vi "Main.vi"(10 "Port Number":i16=4 min=0 max=20, 11 "Module Admin":refnum<class "Delacor_lib_QMH_Module Admin.lvclass">) -> ()   [LabVIEW 2020, in "Ophir Power Meter.lvlib"]
doc: "This template is based off of the Queued Message Handler design pattern and the Queued Message Handler project template that ships with LabVIEW.\n\nThe main difference is that the queue is private to this module and communication between modules is performed via Broadcast and Request events.\n\nRequest events are wrapped in public API methods and are handled in the Event Handling Loop (EHL) of this VI. Any module can register for Broadcast events sent by this module. The EHL generates messages based on user interface actions.\n\nThe Message Handling Loop (MHL) processes messages generated by the EHL, or by other messages. The messages are string values, so new messages can be added easily to the Message Cases case structure in the MHL. Each message cluster can also provide an optional value for Message Data, which is a variant that can be converted to whatever message-specific data is required.\n_____\nBased on Delacor QMH Project Template 5.0.0.82."
uses:
  Ophir Power Meter.lvlib
  <vilib>/Delacor/Delacor QMH/Libraries/Module Admin_class/Delacor_lib_QMH_Module Admin.lvclass
  Module Data--cluster.ctl
  Stop Argument--cluster.ctl
  <vilib>/Delacor/Delacor QMH/Libraries/Message Queue_class/Delacor_lib_QMH_Message Queue.lvclass/Delacor_lib_QMH_Message Queue.ctl
  <vilib>/Delacor/Delacor QMH/Libraries/Module Admin_class/Delacor_lib_QMH_Module Admin.lvclass/Delacor_lib_QMH_Module Admin.ctl
  Get Power Value Argument--cluster.ctl
  Get Power Value (Reply Payload)--cluster.ctl
  Select Range Argument--cluster.ctl
  Get Range Info Argument--cluster.ctl
  Get Range Info (Reply Payload)--cluster.ctl
  <vilib>/Utility/miscctls.llb/LVPointTypeDef.ctl
  <vilib>/Delacor/Delacor QMH/Libraries/Message Queue_class/Delacor_lib_QMH_Enqueue Message (Single).vi
  <vilib>/Delacor/Delacor QMH/Libraries/Module Admin_class/Delacor_lib_QMH_Get External Launch.vi
  <vilib>/Utility/error.llb/Error Cluster From Error Code.vi
  <vilib>/ErrorRing/Error Ring.xnode
  <vilib>/Delacor/Delacor QMH/Libraries/Message Queue_class/Delacor_lib_QMH_Message Queue.lvclass
panel:
  in  "Range":u16(ring)
  out "Power Value":dbl
  out "Units":string
  out "OK ?":bool
  out "Instrument Info":string[](array[string])
  out "error out":errorcluster
  out "Status":string
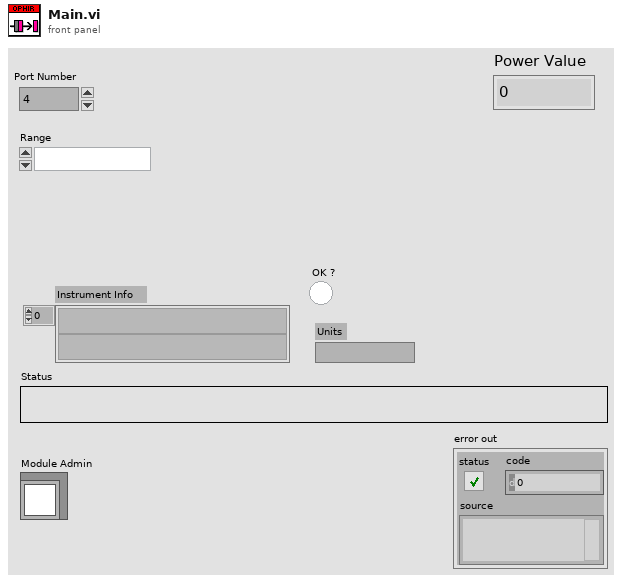
[diagram p1: front panel]
types:
  T1 = typedef "Ophir Power Meter.lvlib/Request Events--cluster.ctl" = cluster{"Stop Module":refnum<user-event>, "Show Panel":refnum<user-event>, "Hide Panel":refnum<user-event>, "Get Module Execution Status":refnum<user-event>, "Show Diagram":refnum<user-event>, "Get Power Value":refnum<user-event>, "Select Range":refnum<user-event>, "Get Range Info":refnum<user-event>}
  T2 = typedef "Ophir Power Meter.lvlib/Module Data--cluster.ctl" = cluster{"Status":string, "Visa Session":refnum<visa-resource-name>, "Range Info":cluster{"Strings Array":string[], "Symbols Array":i32[], "First Index":i32}}
  T3 = enum32{"invalid lock state", "Not Locked", "Locked (No Password)", "Password-protected"}
  T4 = typedef "Ophir Power Meter.lvlib/Stop Argument--cluster.ctl" = cluster{"Origin":string, "Exit via Stop Module Req?":bool, "Wait for Module to stop?":bool}
  T5 = typedef "Ophir Power Meter.lvlib/Get Power Value Argument--cluster.ctl" = cluster{"Wait Notifier":refnum<notifier>, "wait for reply":bool}
  T6 = typedef "Ophir Power Meter.lvlib/Select Range Argument--cluster.ctl" = cluster{"Range Number":i32}
  T7 = typedef "Ophir Power Meter.lvlib/Get Range Info Argument--cluster.ctl" = cluster{"Wait Notifier":refnum<notifier>, "wait for reply":bool}
  T8 = typedef "LVPointTypeDef.ctl" = cluster{"Horizontal":i16, "Vertical":i16}
  T9 = enum32{"Invalid", "Standard", "Closed", "Hidden", "Minimized", "Maximized"}
  T10 = typedef "Ophir Power Meter.lvlib/Get Power Value (Reply Payload)--cluster.ctl" = cluster{"Power Value":dbl, "Get Power Value_error":errorcluster}
  T11 = typedef "Ophir Power Meter.lvlib/Get Range Info (Reply Payload)--cluster.ctl" = cluster{"Range Info":cluster{"Strings Array":string[], "Symbols Array":i32[], "First Index":i32}, "Get Range Info_error":errorcluster}
  T12 = cluster{"Strings Array":string[], "Symbols Array":i32[], "First Index":i32}
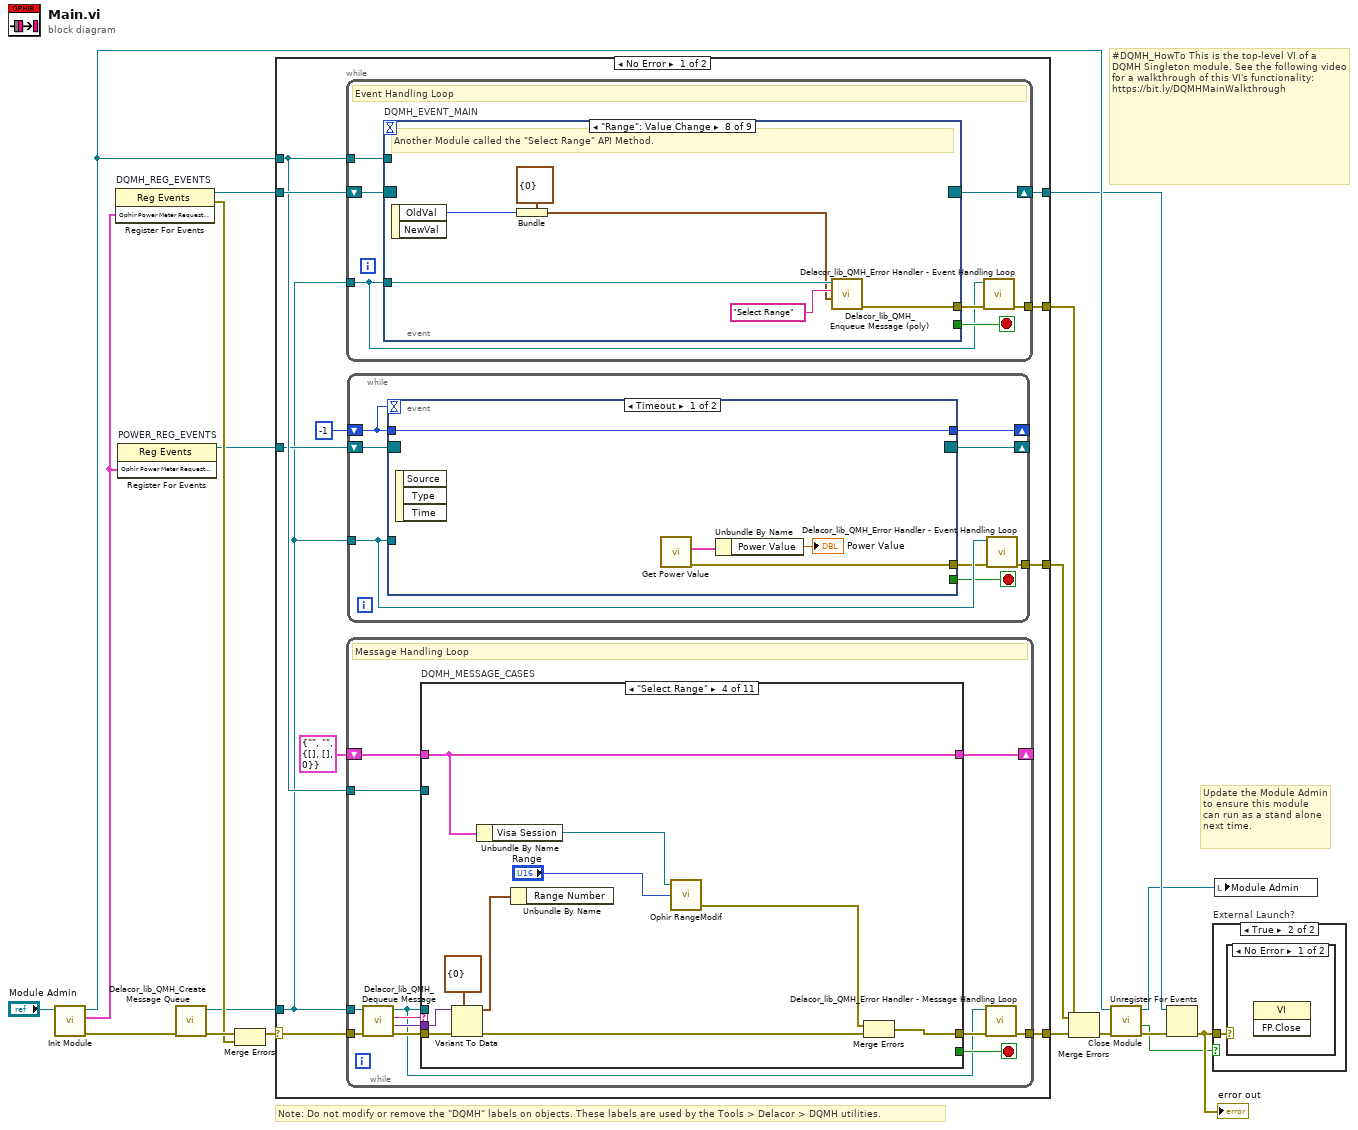
[diagram p0: block diagram]
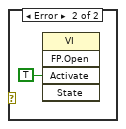
[diagram p3: hidden frame]
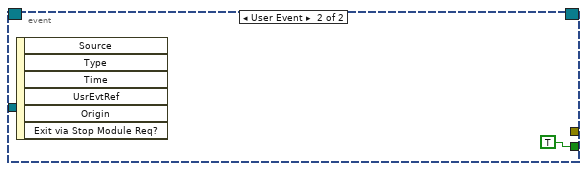
[diagram p4: hidden frame]
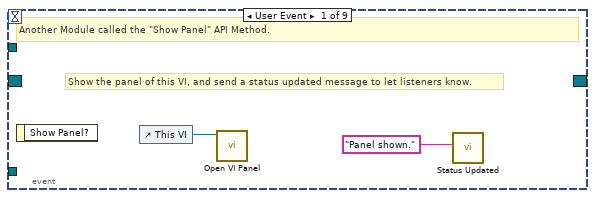
[diagram p5: hidden frame]
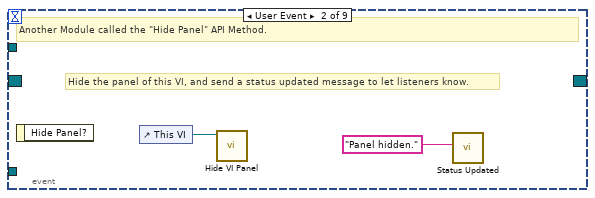
[diagram p6: hidden frame]
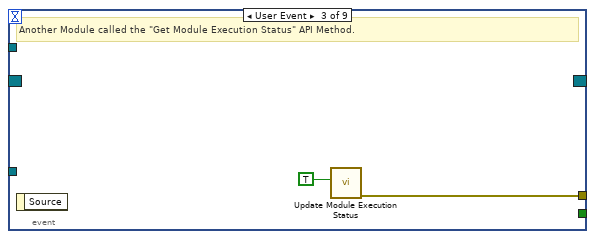
[diagram p7: hidden frame]
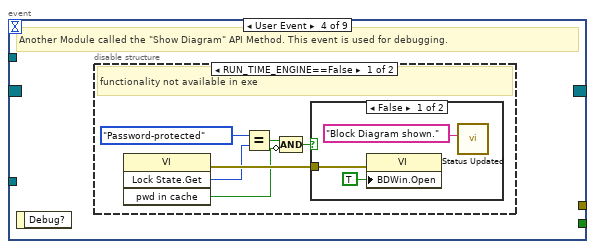
[diagram p8: hidden frame]
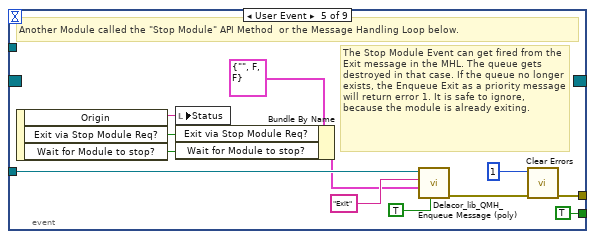
[diagram p11: hidden frame]
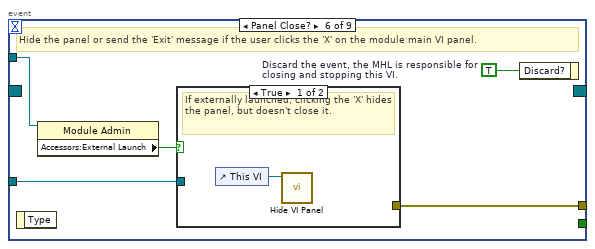
[diagram p12: hidden frame]
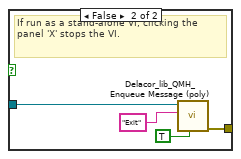
[diagram p13: hidden frame]
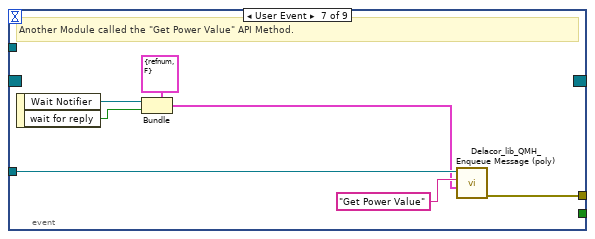
[diagram p14: hidden frame]
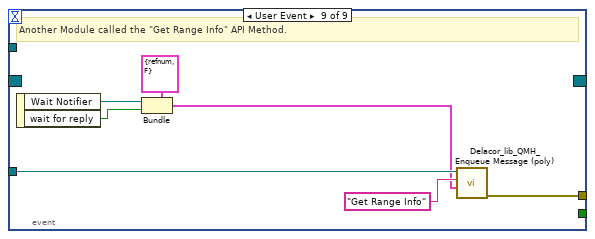
[diagram p15: hidden frame]
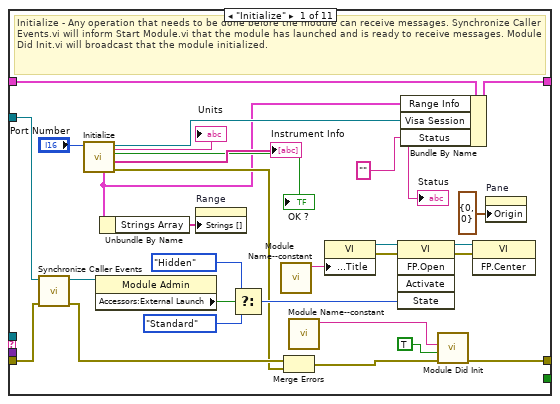
[diagram p16: hidden frame]
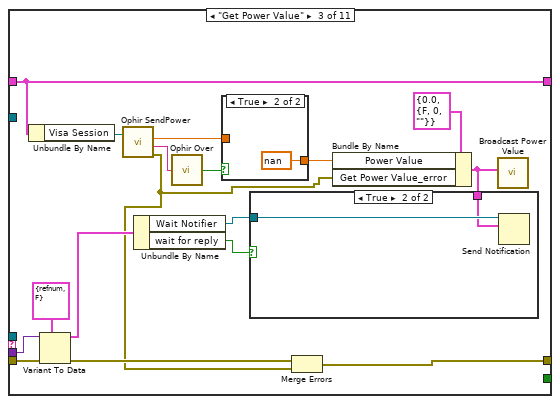
[diagram p18: hidden frame]
diagram:
  # "#DQMH_HowTo This is the top-level VI of a DQMH Singleton module. See the following video for a walkthrough of this VI's functionality: https://bit.ly/DQMHMainWalkthrough"
  # "Note: Do not modify or remove the \"DQMH\" labels on objects. These labels are used by the Tools > Delacor > DQMH utilities."
  # "Update the Module Admin to ensure this module can run as a stand alone next time."
  n1 = call "Init Module.vi"("Singleton Module Admin in"="Module Admin") -> ("error out"=w18:errorcluster, "Ophir Power Meter Request Events"=w3:T1, "Singleton Module Admin out"=w10:refnum<class "Delacor_lib_QMH_Module Admin.lvclass">)  [unwired: 8 in]
  n2 = register-events "DQMH_REG_EVENTS"(w3) -> (reference out=w8:refnum<event-registration>, error out=w11:errorcluster)  [unwired: 2 in]
  n3 = register-events "POWER_REG_EVENTS"(w3) -> (reference out=w2:refnum<event-registration>)  [unwired: 2 in, 1 out]
  n4 = call <vilib>:"Delacor_lib_QMH_Create Message Queue.vi"("error in (no error)"=w18) -> ("error out"=w13:errorcluster, "Message Queue"=w7:refnum<class "Delacor_lib_QMH_Message Queue.lvclass">)  [unwired: 9 in]
  n5 = Merge Errors(w13, w11) -> (w12:errorcluster)
  n6 = case shown="No Error" w12 {
    selector: w12 -> [w28 w270]
    tunnel: [w30 w269] -> w19
    tunnel: [w27 w275] -> w9
    tunnel: w8 -> [w25 w275]
    tunnel: w7 -> [w21 w268]
    tunnel: [w29 _] -> w16
    tunnel: w10 -> [w24 w271]
    tunnel: w2 -> [w23 _]
    tunnel: [w20 _] -> w1
    frame No Error {
      n7 = while {
        tunnel: w21 -> [w44]
        shift-right: [w47] -> w27
        shift-left: w25 -> [w48]
        tunnel: [w49] -> w29
        tunnel: w24 -> [w45]
        stop <- w46 stop-if-true
        # "Event Handling Loop"
        n8 = event "DQMH_EVENT_MAIN" shown="[7] \"Range\": Value Change" {
          selector: w48 -> [_ _ _ _ _ _ _ _ _]
          dyn-events: [_ _ _ _ _ _ _ _ _] -> w47
          timeout: _ -> [_ _ _ _ _ _ _ _ _]
          tunnel: [_ _ _ _ TRUE ("Discard?") _ _ _ _] -> w46
          tunnel: w44 -> [_ _ _ _ w73 w80 w94 w100 w107]
          tunnel: [_ _ w56 _ w76 w82 w88 w95 w101] -> w50
          tunnel: w45 -> [_ _ _ _ _ w79 _ _ _]
          event User Event {
            # "Show the panel of this VI, and send a status updated message to let listeners know."
            # "Another Module called the \"Show Panel\" API Method."
            n9 = event-data() -> ()  [unwired: 1 in, 1 out]
            n10 = control-ref of="This VI"() -> (w52:refnum<vi>)
            n11 = call "Open VI Panel.vi"("VI"=w52) -> ()  [unwired: 10 in, 1 out]
            n12 = call "Status Updated.vi"("Status"="Panel shown." ("format string")) -> ()  [unwired: 10 in, 1 out]
          }
          event User Event {
            # "Hide the panel of this VI, and send a status updated message to let listeners know."
            # "Another Module called the \"Hide Panel\" API Method."
            n13 = event-data() -> ()  [unwired: 1 in, 1 out]
            n14 = control-ref of="This VI"() -> (w54:refnum<vi>)
            n15 = call "Hide VI Panel.vi"("VI"=w54) -> ()  [unwired: 10 in, 1 out]
            n16 = call "Status Updated.vi"("Status"="Panel hidden." ("format string")) -> ()  [unwired: 10 in, 1 out]
          }
          event User Event {
            # "Another Module called the \"Get Module Execution Status\" API Method."
            n17 = event-data() -> ()  [unwired: 1 in, 1 out]
            n18 = call "Update Module Execution Status.vi"("Running?"=TRUE) -> ("error out"=w56:errorcluster)  [unwired: 10 in]
          }
          event User Event {
            # "Another Module called the \"Show Diagram\" API Method. This event is used for debugging."
            n19 = event-data() -> ()  [unwired: 1 in, 1 out]
            n20 = disable-structure shown="RUN_TIME_ENGINE==False" {
              frame condition #0 (active) {
                # "functionality not available in exe"
                n21 = invoke class="VI" method="Lock State.Get"() -> (error out=w62:errorcluster, "Get Lock State"=w61:T3, "pwd in cache"=w58:bool)  [unwired: 4 in, 1 out]
                n22 = Equal?(x=T3."Password-protected", y=w61) -> (x = y?=w59:bool)
                n23 = Compound Arithmetic op=AND(w59, invert w58) -> (w57:bool)
                n24 = case shown="False" w57 {
                  tunnel: w62 -> [w65 _]
                  frame False {
                    n25 = property class="VI"(error in=w65, "BDWin.Open"=TRUE ("Block Diagram Window:Open")) -> ()  [unwired: 1 in, 2 out]
                    n26 = call "Status Updated.vi"("Status"="Block Diagram shown." ("format string")) -> ()  [unwired: 10 in, 1 out]
                  }
                  frame True {
                    # "Password-protected VI, and the password is not in the cache. Do not show the diagram."
                  }
                }
              }
              frame condition #1 {
              }
            }
          }
          event User Event {
            # "The Stop Module Event can get fired from the Exit message in the MHL. The queue gets destroyed in that case. If the queue no longer exists, the Enqueue Exit as a priority message will return error 1. It is safe to ignore, because the module is already exiting."
            # "Another Module called the \"Stop Module\" API Method  or the Message Handling Loop below."
            n27 = event-data() -> ("Origin"=w72:string, "Exit via Stop Module Req?"=w68:bool, "Wait for Module to stop?"=w67:bool)  [unwired: 1 in]
            n28 = local write "Status"(w72) -> ()
            n29 = Bundle By Name(cluster=T4 {"Origin"="", "Exit via Stop Module Req?"=FALSE, "Wait for Module to stop?"=FALSE} ("Stop Argument"), "Exit via Stop Module Req?"=w68, "Wait for Module to stop?"=w67) -> (w66:T4)
            n30 = call-poly <vilib>:"Delacor_lib_QMH_Enqueue Message (poly).vi"("Priority Message? (F)"=TRUE, "Message Data"=w66, "Message"="Exit", "Message Queue in"=w73) -> ("error out"=w77:errorcluster)  [unwired: 6 in, 1 out]
            n31 = call <vilib>:"Clear Errors.vi"("error in (no error)"=w77, "specific error code to clear (0: all)"=1) -> ("error out"=w76:errorcluster)  [unwired: 4 in, 1 out]
          }
          event Panel Close? {
            w81 = TRUE  # Discard the event, the MHL is responsible for closing and stopping this VI.
            # "Hide the panel or send the 'Exit' message if the user clicks the 'X' on the module main VI panel."
            n32 = event-data() -> ()  [unwired: 1 in, 1 out]
            n33 = property class="Module Admin"(reference=w79) -> ("Accessors:External Launch"=w78:bool)  [unwired: 1 in, 2 out]
            n34 = case shown="True" w78 {
              tunnel: w80 -> [_ w86]
              tunnel: [_ w87] -> w82
              frame True {
                # "If externally launched, clicking the 'X' hides the panel, but doesn't close it."
                n35 = control-ref of="This VI"() -> (w83:refnum<vi>)
                n36 = call "Hide VI Panel.vi"("VI"=w83) -> ()  [unwired: 10 in, 1 out]
              }
              frame False {
                # "If run as a stand-alone VI, clicking the panel 'X' stops the VI."
                n37 = call-poly <vilib>:"Delacor_lib_QMH_Enqueue Message (poly).vi"("Priority Message? (F)"=TRUE, "Message"="Exit", "Message Queue in"=w86) -> ("error out"=w87:errorcluster)  [unwired: 7 in, 1 out]
              }
            }
            n38 = event-data("Discard?"=w81) -> ()  [unwired: 1 in, 1 out]
          }
          event User Event {
            # "Another Module called the \"Get Power Value\" API Method."
            n39 = event-data() -> ("Wait Notifier"=w90:refnum<notifier>, "wait for reply"=w89:bool)  [unwired: 1 in]
            n40 = Bundle(cluster=T5 {"Wait Notifier"=refnum, "wait for reply"=FALSE} ("Get Power Value Argument"), "Wait Notifier"=w90, "wait for reply"=w89) -> (w91:T5)
            n41 = call-poly <vilib>:"Delacor_lib_QMH_Enqueue Message (poly).vi"("Message Data"=w91, "Message"="Get Power Value", "Message Queue in"=w94) -> ("error out"=w88:errorcluster)  [unwired: 7 in, 1 out]
          }
          event "Range": Value Change {
            # "Another Module called the \"Select Range\" API Method."
            n42 = event-data() -> ("OldVal"=w96:u16)  [unwired: 1 in, 1 out]
            n43 = Bundle(cluster=T6 {"Range Number"=0} ("Select Range Argument"), "Range Number"=w96) -> (w97:T6)
            n44 = call-poly <vilib>:"Delacor_lib_QMH_Enqueue Message (poly).vi"("Message Data"=w97, "Message"="Select Range", "Message Queue in"=w100) -> ("error out"=w95:errorcluster)  [unwired: 7 in, 1 out]
          }
          event User Event {
            # "Another Module called the \"Get Range Info\" API Method."
            n45 = event-data() -> ("Wait Notifier"=w103:refnum<notifier>, "wait for reply"=w102:bool)  [unwired: 1 in]
            n46 = Bundle(cluster=T7 {"Wait Notifier"=refnum, "wait for reply"=FALSE} ("Get Range Info Argument"), "Wait Notifier"=w103, "wait for reply"=w102) -> (w104:T7)
            n47 = call-poly <vilib>:"Delacor_lib_QMH_Enqueue Message (poly).vi"("Message Data"=w104, "Message"="Get Range Info", "Message Queue in"=w107) -> ("error out"=w101:errorcluster)  [unwired: 7 in, 1 out]
          }
        }
        n48 = call-dynamic "Delacor_lib_QMH_Error Handler - Event Handling Loop.vi"("error in (no error)"=w50, "Message Queue in"=w44) -> ("dup error in"=w49:errorcluster)  [unwired: 8 in, 1 out]
      }
      n49 = while {
        tunnel: w21 -> [w110]
        shift-right: [w114] -> _
        shift-left: T2 {"Status"="", "Visa Session"="", "Range Info"={"Strings Array"=[], "Symbols Array"=[], "First Index"=0}} ("Data Cluster") -> [w115]
        tunnel: w28 -> [w118]
        tunnel: [w116] -> w30
        tunnel: w24 -> [w108]
        stop <- w113 stop-if-true
        # "Message Handling Loop"
        n50 = call-dynamic "Delacor_lib_QMH_Dequeue Message.vi"("error in (no error)"=w118, "Message Queue in"=w110) -> ("error out"=w117:errorcluster, "Message Data"=w111:variant, "Message"=w112:string, "Message Queue out"=w109:refnum<class "Delacor_lib_QMH_Message Queue.lvclass">)  [unwired: 6 in]
        n51 = case "DQMH_MESSAGE_CASES" shown="\"Select Range\"" w112 {
          selector: w112 -> [_ _ _ _ _ _ _ _ _ _ w255]
          tunnel: w109 -> [_ _ _ _ _ _ _ _ w222 w247 _]
          tunnel: w117 -> [w146 w150 w167 w181 w199 w204 w206 w211 w229 w253 w257]
          tunnel: [w144 w150 w158 w176 w190 w203 w206 w210 w225 w250 w258] -> w119
          tunnel: w115 -> [w135 w149 w157 w174 w189 w202 w205 w208 w224 w239 w256]
          tunnel: [w134 w149 w157 w174 w183 w202 w205 w208 w224 w239 w256] -> w114
          tunnel: [_ _ _ _ _ _ _ _ _ w246 _] -> w113
          tunnel: w111 -> [_ _ w165 w179 w197 _ _ _ w223 w245 _]
          tunnel: w108 -> [w136 _ _ _ _ _ _ _ w221 w240 _]
          frame "Initialize" {
            w125 = "" ("Status")
            # "Initialize - Any operation that needs to be done before the module can receive messages. Synchronize Caller Events.vi will inform Start Module.vi that the module has launched and is ready to receive messages. Module Did Init.vi will broadcast that the module initialized."
            n52 = call "Synchronize Caller Events.vi"("error in (no error)"=w146, "Singleton Module Admin in"=w136) -> ("error out"=w145:errorcluster, "Singleton Module Admin out"=w131:refnum<class "Delacor_lib_QMH_Module Admin.lvclass">)  [unwired: 8 in]
            n53 = call "Initialize.vi"("Port Number"="Port Number") -> ("error out"=w127:errorcluster, "Instrument Info"=→"Instrument Info":string[], "OK ?"=→"OK ?":bool, "Visa Session"=w122:refnum<visa-resource-name>, "Range Info"=w121:T12, "Units"=→"Units":string)  [unwired: 5 in]
            n54 = property class="Module Admin"(reference=w131) -> ("Accessors:External Launch"=w140:bool)  [unwired: 1 in, 2 out]
            n55 = Unbundle By Name(w121) -> ("Strings Array"=w120:string[])
            n56 = property on="Range" class="Ring (strict)"("Strings []"=w120) -> ()  [unwired: 2 in, 2 out]
            n57 = Select(t=T9."Hidden" ("State"), s=w140, f=T9."Standard" ("State")) -> (s? t:f=w137:T9)
            n58 = call "Module Name--constant.vi"() -> ("Module Name"=w143:string)  [unwired: 11 in]
            n59 = Merge Errors(w145, w127) -> (w128:errorcluster)
            n60 = call "Module Name--constant.vi"() -> ("Module Name"=w132:string)  [unwired: 11 in]
            n61 = property class="VI"("Front Panel.Title"=w143) -> (reference out=w142:refnum<vi>, error out=w148:errorcluster)  [unwired: 2 in]
            n62 = invoke class="VI" method="FP.Open"(reference=w142, error in=w148, "State"=w137) -> (reference out=w141:refnum<vi>, error out=w147:errorcluster)  [unwired: 2 in, 3 out]
            n63 = Bundle By Name(cluster=w135, "Range Info"=w121, "Visa Session"=w122, "Status"=w125) -> (w134:T2)
            n64 = call "Module Did Init.vi"("error in (no error)"=w128, "Initialized?"=TRUE, "Origin"=w132) -> ("error out"=w144:errorcluster)  [unwired: 8 in]
            n65 = invoke class="VI" method="FP.Center"(reference=w141, error in=w147) -> ()  [unwired: 1 in, 3 out]
            n66 = property on="Pane" class="Pane"("Origin"=T8 {"Horizontal"=0, "Vertical"=0}) -> ()  [unwired: 2 in, 2 out]
            "Status" <- w125
          }
          frame "--- Module Specific ---" {
            # "Separator -- The following cases handle messages specific to this Module."
          }
          frame "Get Power Value" {
            n67 = Unbundle By Name(w157) -> ("Visa Session"=w156:refnum<visa-resource-name>)
            n68 = Variant To Data(error in=w167, type=T5 {"Wait Notifier"=refnum, "wait for reply"=FALSE} ("Get Power Value Argument"), Variant=w165) -> (data=w163:T5, error out=w166:errorcluster)
            n69 = call <instrlib>:"Ophir SendPower.vi"("Visa Session"=w156) -> ("Value Number"=w152:dbl, "Value String"=w155:string, "error out"=w151:errorcluster)  [unwired: 1 in, 1 out]
            n70 = Unbundle By Name(w163) -> ("Wait Notifier"=w162:refnum<notifier>, "wait for reply"=w161:bool)
            n71 = call <instrlib>:"Ophir Over.vi"("Value String"=w155) -> ("Overrange"=w154:bool)
            n72 = case shown="True" w154 {
              tunnel: [w168 nan ("Value Number")] -> w153
              tunnel: w152 -> [w168 _]
              frame False {
              }
              frame True {
              }
            }
            n73 = Merge Errors(w166, w151) -> (w158:errorcluster)
            n74 = Bundle By Name(cluster=T10 {"Power Value"=0.0, "Get Power Value_error"={"status"=FALSE, "code"=0, "source"=""}} ("Get Power Value (Reply Payload)"), "Power Value"=w153, "Get Power Value_error"=w151) -> (w160:T10)
            n75 = case shown="True" w161 {
              tunnel: w162 -> [_ w171]
              tunnel: w160 -> [_ w170]
              frame False {
              }
              frame True {
                n76 = Send Notification(notification=w170, notifier=w171) -> ()  [unwired: 1 in, 2 out]
              }
            }
            n77 = call "Broadcast Power Value.vi"("Reply Payload"=w160) -> ()  [unwired: 10 in, 1 out]
          }
          frame "Select Range" {
            n78 = Variant To Data(error in=w181, type=T6 {"Range Number"=0} ("Select Range Argument"), Variant=w179) -> (data=w177:T6, error out=w180:errorcluster)
            n79 = Unbundle By Name(w174) -> ("Visa Session"=w173:refnum<visa-resource-name>)
            n80 = Unbundle By Name(w177) -> ()  [unwired: 1 out]
            n81 = call <instrlib>:"Ophir RangeModif.vi"("Range Number(0)"="Range", "Visa Session"=w173) -> ("error out"=w175:errorcluster)  [unwired: 1 in, 2 out]
            n82 = Merge Errors(w175, w180) -> (w176:errorcluster)
          }
          frame "Get Range Info" {
            n83 = Variant To Data(error in=w199, type=T7 {"Wait Notifier"=refnum, "wait for reply"=FALSE} ("Get Range Info Argument"), Variant=w197) -> (data=w195:T7, error out=w198:errorcluster)
            n84 = Unbundle By Name(w189) -> ("Visa Session"=w188:refnum<visa-resource-name>)
            n85 = Unbundle By Name(w195) -> ("Wait Notifier"=w194:refnum<notifier>, "wait for reply"=w193:bool)
            n86 = call <instrlib>:"Ophir RangeList.vi"("Visa Session"=w188) -> ("error out"=w184:errorcluster, "Strings Array"=w187:string[], "Symbols Array"=w186:i32[], "First Index"=w185:i32)  [unwired: 2 in, 1 out]
            n87 = Bundle("Strings Array"=w187, "Symbols Array"=w186, "First Index"=w185) -> (w182:T12)  [unwired: 1 in]
            n88 = Bundle By Name(cluster=T11 {"Range Info"={"Strings Array"=[], "Symbols Array"=[], "First Index"=0}, "Get Range Info_error"={"status"=FALSE, "code"=0, "source"=""}} ("Get Range Info (Reply Payload)"), "Range Info"=w182, "Get Range Info_error"=w184) -> (w192:T11)
            n89 = case shown="True" w193 {
              tunnel: w194 -> [_ w201]
              tunnel: w192 -> [_ w200]
              frame False {
              }
              frame True {
                n90 = Send Notification(notification=w200, notifier=w201) -> ()  [unwired: 1 in, 2 out]
              }
            }
            n91 = Merge Errors(w198, w184) -> (w190:errorcluster)
            n92 = Bundle By Name(cluster=w189, "Range Info"=w182) -> (w183:T2)
          }
          frame "---Copy This Frame---" {
            # "Duplicate this frame when creating new messages.  Change this comment in the duplicated frame to describe this message."
            n93 = Merge Errors(w204) -> (w203:errorcluster)
          }
          frame "--- Exit and Error Handling---" {
            # "Separator - The following cases handle errors and exit messages."
          }
          frame "Simulate MHL Error" {
            # "#DQMH_HowTo The 'Simulate MHL Error' button  illustrates how the MHL handles errors. This event is instructional in nature and can be removed."
            # "Simulate an error occurring at the MHL"
            n94 = call "Module Name--constant.vi"() -> ("Module Name"=w207:string)  [unwired: 11 in]
            n95 = xnode "Error Ring"("parameter 0"=w207) -> ("error out"=w209:errorcluster)
            n96 = Merge Errors(w211, w209) -> (w210:errorcluster)
          }
          frame "Error" {
            # "#CodeRecommended - If you ever change the name of this \"Error\" message, you'll need to update the name in the Check Loop Error.vi as well."
            # "#CodeRecommended - If the module is running in standalone mode (External Launch = FALSE), this code will pop up an error dialog and call the 'Exit' message if an error occurs. Add more fine-grained error handling here."
            # "Error - Check the error message data and respond accordingly. This message is sent by the \"Error Handler\" VIs at the end of each loop in this application."
            n97 = property class="Module Admin"(reference=w221) -> ("Accessors:External Launch"=w220:bool)  [unwired: 1 in, 2 out]
            n98 = Variant To Data(error in=w229, type=errorcluster {"status"=FALSE, "code"=0, "source"=""} ("error constant"), Variant=w223) -> (data=w230:errorcluster, error out=w227:errorcluster)
            n99 = call "Module Name--constant.vi"() -> ("Module Name"=w219:string)  [unwired: 11 in]
            n100 = call "Error Reported.vi"("Additional Information"=w219, "Error"=w230) -> ()  [unwired: 9 in, 1 out]
            n101 = case shown="False" w220 {
              tunnel: [w236 _] -> w226
              tunnel: w222 -> [w234 _]
              tunnel: w230 -> [w235 _]
              frame False {
                n102 = call <vilib>:"Simple Error Handler.vi"("error in (no error)"=w235) -> ("error out"=w231:errorcluster)  [unwired: 4 in, 4 out]
                n103 = call-poly <vilib>:"Delacor_lib_QMH_Enqueue Message (poly).vi"("Priority Message? (F)"=TRUE, "Message"="Exit", "Message Queue in"=w234) -> ("error out"=w236:errorcluster)  [unwired: 7 in, 1 out]
                n104 = call <instrlib>:"Ophir Error Message.vi"("error in (no error)"=w231) -> ()  [unwired: 3 in, 4 out]
              }
              frame True {
                # "If the module was launched externally, calling the Error Reported broadcast VI is the only action performed by the \"Error\" message. The module's caller can then process the error appropriately."
              }
            }
            n105 = Merge Errors(w227, w226) -> (w225:errorcluster)
            n106 = local write "error out"(w225) -> ()
          }
          frame "Exit" {
            w244 = 91  # 91: not all Exit messages will have an argument
            w246 = TRUE  # Stop the VI
            # "Release the message queue reference"
            # "Exit - Exit the application."
            n107 = Variant To Data(error in=w253, type=T4 {"Origin"="", "Exit via Stop Module Req?"=FALSE, "Wait for Module to stop?"=FALSE} ("Stop Argument"), Variant=w245) -> (data=w242:T4, error out=w249:errorcluster)
            n108 = Unbundle By Name(w239) -> ("Visa Session"=w238:refnum<visa-resource-name>)
            n109 = call <vilib>:"Clear Errors.vi"("error in (no error)"=w249, "specific error code to clear (0: all)"=w244) -> ("error out"=w252:errorcluster)  [unwired: 4 in, 1 out]
            n110 = VISA Close(VISA resource name=w238) -> (error out=w237:errorcluster)  [unwired: 1 in]
            n111 = control-ref of="This VI"() -> (w241:refnum<vi>)
            n112 = call <instrlib>:"Ophir Error Message.vi"("error in (no error)"=w237) -> ()  [unwired: 3 in, 4 out]
            n113 = call-dynamic "Delacor_lib_QMH_Release Message Queue.vi"("error in (no error)"=w252, "Message Queue"=w247) -> ("error out"=w251:errorcluster)  [unwired: 9 in]
            n114 = call "Handle Exit.vi"("Stop Argument"=w242, "Admin in"=w240, "VI reference"=w241) -> ("error out"=w248:errorcluster)  [unwired: 7 in, 1 out]
            n115 = Merge Errors(w237, w251, w248) -> (w250:errorcluster)
          }
          frame Default {
            # "'Default' case only runs if there is a message that isn't defined in any of the other cases.  Output a programming error."
            n116 = call "Module Name--constant.vi"() -> ("Module Name"=w254:string)  [unwired: 11 in]
            n117 = xnode "Error Ring"("parameter 0"=w255, "parameter 1"=w254) -> ("error out"=w259:errorcluster)
            n118 = Merge Errors(w257, w259) -> (w258:errorcluster)
          }
        }
        n119 = call-dynamic "Delacor_lib_QMH_Error Handler - Message Handling Loop.vi"("error in (no error)"=w119, "Message Queue in"=w109) -> ("dup error in"=w116:errorcluster)  [unwired: 8 in, 1 out]
      }
      n120 = while {
        shift-right: [w35] -> _
        shift-left: w23 -> [w38]
        shift-right: [w36] -> _
        shift-left: -1 -> [w37]
        tunnel: w21 -> [w34]
        tunnel: [w33] -> w20
        stop <- w32 stop-if-true
        n121 = event shown="[0] Timeout" {
          selector: w38 -> [_ _]
          dyn-events: [_ _] -> w35
          timeout: w37 -> [_ _]
          tunnel: w37 -> [w42 _]
          tunnel: [w42 _] -> w36
          tunnel: w34 -> [_ _]
          tunnel: [_ TRUE] -> w32
          tunnel: [w41 _] -> w31
          event Timeout {
            n122 = event-data() -> ()  [unwired: 1 in, 3 out]
            n123 = call "Get Power Value.vi"() -> ("error out"=w41:errorcluster, "Reply Payload"=w40:T10)  [unwired: 9 in, 1 out]
            n124 = Unbundle By Name(w40) -> ("Power Value"=→"Power Value":dbl)
          }
          event User Event {
            n125 = event-data() -> ()  [unwired: 1 in, 6 out]
          }
        }
        n126 = call-dynamic "Delacor_lib_QMH_Error Handler - Event Handling Loop.vi"("error in (no error)"=w31, "Message Queue in"=w34) -> ("dup error in"=w33:errorcluster)  [unwired: 8 in, 1 out]
      }
    }
    frame Error {
      # "Synchronize Caller Events.vi will inform Start Module.vi that the module has launched and will let the code calling Start Module.vi register for broadcasts and would permit the caller receive the broadcast that an error occurred at launch time."
      n127 = call-dynamic "Delacor_lib_QMH_Release Message Queue.vi"("error in (no error)"=w270, "Message Queue"=w268) -> ("error out"=w269:errorcluster)  [unwired: 9 in]
      n128 = call "Synchronize Caller Events.vi"("Singleton Module Admin in"=w271) -> ("error out"=w276:errorcluster)  [unwired: 9 in, 1 out]
      n129 = call "Module Name--constant.vi"() -> ("Module Name"=w274:string)  [unwired: 11 in]
      n130 = Format Into String(format string="An error occurred during initialization. %s is no longer running.", w274) -> (resulting string=w272:string)  [unwired: 2 in, 1 out]
      n131 = Merge Errors(w269, w276) -> (w277:errorcluster)
      n132 = call "Error Reported.vi"("Additional Information"=w272, "Error"=w277) -> ()  [unwired: 9 in, 1 out]
    }
  }
  n133 = Merge Errors(w1, w16, w19) -> (w15:errorcluster)
  n134 = call "Close Module.vi"("error in (no error)"=w15, "Module Admin in"=w10) -> ("error out"=w17:errorcluster, "External Launch"=w4:bool, "Module Admin out"=w5:refnum<class "Delacor_lib_QMH_Module Admin.lvclass">)  [unwired: 7 in]
  n135 = Unregister For Events(event registration refnum=w9, error in=w17) -> (error out=w14:errorcluster)
  "error out" <- w14
  n136 = case "External Launch?" shown="True" w4 {
    tunnel: w14 -> [_ w278]
    frame False {
    }
    frame True {
      n137 = case shown="No Error" w278 {
        frame No Error {
          n138 = invoke class="VI" method="FP.Close"() -> ()  [unwired: 3 in, 3 out]
        }
        frame Error {
          n139 = invoke class="VI" method="FP.Open"("Activate"=TRUE ("Activate?")) -> ()  [unwired: 4 in, 5 out]
        }
      }
    }
  }
  n140 = local write "Module Admin"(w5) -> ()
